vi "2 RIO.vi"   [LabVIEW 2011]
uses:
  2 Globals/2 Global.vi
types:
  T1 = typedef "UTM Location.ctl" = cluster{"UTM Zone":dbl, "Hemisphere":enum16{"North", "South"}, "East":dbl, "North":dbl}
  T2 = typedef "Velocity.ctl" = cluster{"East":dbl, "North":dbl}
  T3 = typedef "apparent wind direction.ctl" = dbl
  T4 = typedef "sail setpt.ctl" = dbl
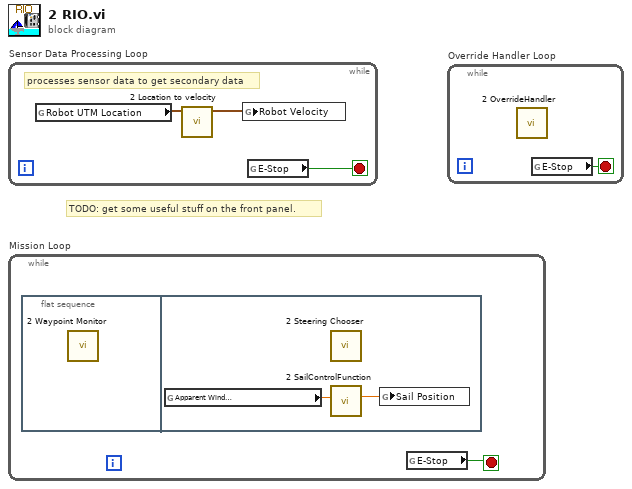
[diagram p0: block diagram]
diagram:
  # "TODO: get some useful stuff on the front panel."
  n1 = while "Sensor Data Processing Loop" {
    stop <- w1 stop-if-true
    # "processes sensor data to get secondary data"
    n2 = global read "2 Global.vi" "Robot UTM Location"() -> (w2:T1)
    n3 = call "2 Location to velocity.vi"("Robot UTM Location"=w2) -> ("Velocity"=w3:T2)  [unwired: 10 in]
    n4 = global write "2 Global.vi" "Robot Velocity"(w3) -> ()
    n5 = global read "2 Global.vi" "E-Stop"() -> (w1:bool)
  }
  n6 = while "Mission Loop" {
    stop <- w4 stop-if-true
    n7 = flat-sequence {
      frame #0 {
        n8 = call "2 Waypoint Monitor.vi"() -> ()  [unwired: 12 in]
      }
      frame #1 {
        n9 = global read "2 Global.vi" "Apparent Wind\nDirection"() -> (w6:T3)
        n10 = call "2 Steering Chooser.vi"() -> ()  [unwired: 12 in]
        n11 = call "2 SailControlFunction.vi"("Apparent Wind\nDirection"=w6) -> ("Sail Position"=w5:T4)  [unwired: 10 in]
        n12 = global write "2 Global.vi" "Sail Position"(w5) -> ()
      }
    }
    n13 = global read "2 Global.vi" "E-Stop"() -> (w4:bool)
  }
  n14 = while "Override Handler Loop" {
    stop <- w7 stop-if-true
    n15 = call "2 OverrideHandler.vi"() -> ()  [unwired: 12 in]
    n16 = global read "2 Global.vi" "E-Stop"() -> (w7:bool)
  }
